vi "Validate Return.vi"(8 "error in":errorcluster, 9 "Divisor":i32, 10 "Rtn Str":string) -> (0 "error out":errorcluster, 1 "outputStr":string, 2 "Output Value":sgl)   [LabVIEW 2015, in "TE Cooler.lvlib" / "TE Cooler.lvclass"]
doc: "Check the return of the controller. From the manual:\n\nIf the temperature controller receives the query and the checksum is correct, the temperature controller will respond by sending back a “return value” and the checksum of those eight ASCII characters:\n(stx)DDDDDDDDSS(ack)\nIf the checksum for a command or query is not correct the temperature controller will respond with eight upper case X’s and then c0, which is the checksum of these eight X’s:\n(stx)XXXXXXXXc0(ack)"
uses:
  TE Cooler.lvclass
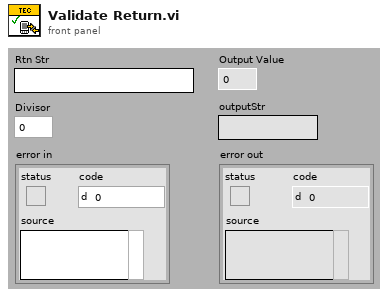
[diagram p1: front panel]
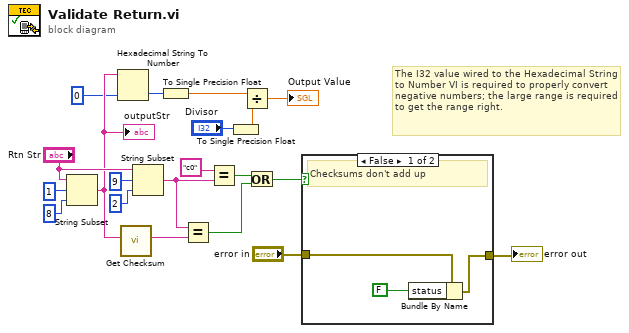
[diagram p0: block diagram]
diagram:
  # "The I32 value wired to the Hexadecimal String to Number VI is required to properly convert negative numbers; the large range is required to get the range right."
  n1 = String Subset(string="Rtn Str", offset (0)=1 ("length (rest)"), length (rest)=8 ("length (rest)")) -> (substring=w12:string)
  "outputStr" <- w12
  n2 = Hexadecimal String To Number(string=w12, default (0uL)=0 ("default (0 U32)")) -> (number=w3:i32)  [unwired: 2 out]
  n3 = call "Get Checksum.vi"("Input"=w12) -> ("Checksum"=w14:string)  [unwired: 10 in]
  n4 = String Subset(string="Rtn Str", offset (0)=9, length (rest)=2 ("length (rest)")) -> (substring=w9:string)
  n5 = To Single Precision Float(number=w3) -> (single precision float=w2:sgl)
  n6 = Equal?(x=w9, y=w14) -> (x = y?=w10:bool)
  n7 = Equal?(x="c0", y=w9) -> (x = y?=w7:bool)
  n8 = To Single Precision Float(number="Divisor") -> (single precision float=w4:sgl)
  n9 = Divide(x=w2, y=w4) -> (x/y=→"Output Value":sgl)
  n10 = Or(x=w7, y=w10) -> (x .or. y?=w6:bool)
  n11 = case shown="False" w6 {
    tunnel: [w21 w24] -> w19
    tunnel: "error in" -> [w23 w24]
    frame False {
      # "Checksums don't add up"
      n12 = Bundle By Name(cluster=w23, "status"=FALSE) -> (w21:errorcluster)
    }
    frame True {
    }
  }
  "error out" <- w19
